vi "Calculate threat.vi"(8 "error in (no error)":errorcluster, 11 "Position in":refnum<class "Position.lvclass">) -> (0 "error out":errorcluster, 2 "Threatened squares":T1[](array[typedef]), 3 "Position out":refnum<class "Position.lvclass">)   [LabVIEW 2016, in "Chesslib.lvlib" / "Position.lvclass"]
uses:
  Position.lvclass
  Moves/Move/Move.lvclass
  typedef/Rank.ctl
  Chesslib.lvlib
  typedef/File.ctl
  typedef/Square.ctl
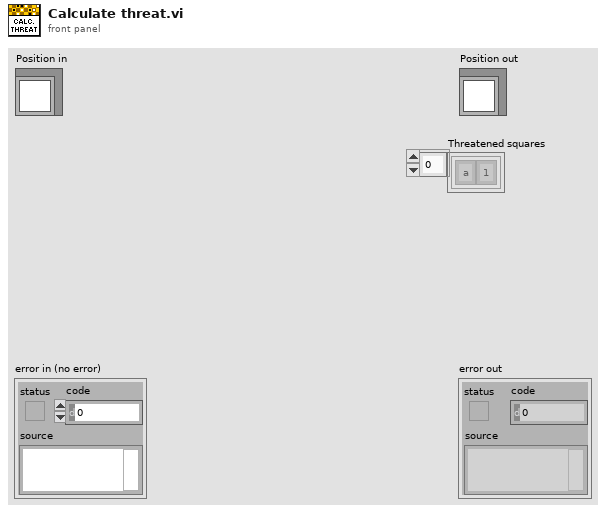
[diagram p1: front panel]
types:
  T1 = typedef "Chesslib.lvlib/Square.ctl" = cluster{"File":T2, "Rank":T3}
  T2 = typedef "Chesslib.lvlib/File.ctl" = enum8{"a", "b", "c", "d", "e", "f", "g", "h"}
  T3 = typedef "Chesslib.lvlib/Rank.ctl" = enum8{"1", "2", "3", "4", "5", "6", "7", "8"}
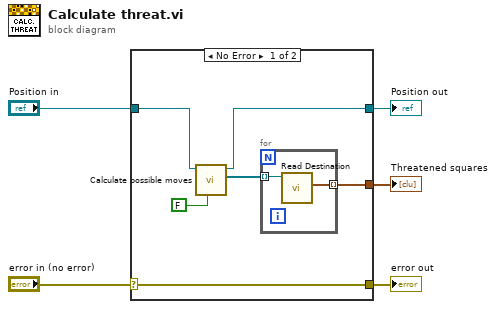
[diagram p0: block diagram]
diagram:
  n1 = case shown="No Error" "error in (no error)" {
    selector: "error in (no error)" -> [w11 w15]
    tunnel: [w11 w15] -> w4
    tunnel: [w8 w14] -> w2
    tunnel: "Position in" -> [w9 w14]
    tunnel: [w10 _] -> w1
    frame No Error {
      n2 = call "Calculate possible moves.vi"("Prune checked moves (T)"=FALSE, "Position in"=w9) -> ("Moves"=w7:refnum<class "Move.lvclass">[], "Position out"=w8:refnum<class "Position.lvclass">)  [unwired: 7 in, 1 out]
      n3 = for {
        tunnel: w7 -> [w13] mode=indexing
        tunnel: [w12] -> w10 mode=indexing
        n4 = call "Read Destination.vi"("Move in"=w13) -> ("Square"=w12:T1)  [unwired: 9 in, 1 out]
      }
    }
    frame Error {
    }
  }
  "error out" <- w4
  "Position out" <- w2
  "Threatened squares" <- w1
